vi "Init.vi"(8 "error in (no error)":errorcluster, 11 "reference in":refnum<class "Test_Base.lvclass">) -> (0 "error out":errorcluster, 3 "reference out":refnum<class "Test_Base.lvclass">)   [LabVIEW 2022 SP3, in "Test_Base.lvlib" / "Test_Base.lvclass"]
uses:
  Test_Base.lvclass
  Components/ViPER.lvlibp/ViPER.lvclass
  Components/TestView_Base.lvlibp/TestView_Base.lvclass
  Components/MES_Base.lvlibp/MES_Base.lvclass
  C:/Projects/Medulla/ViPER/Examples/Flux_Capacitor_Tester/Components/ViPER.lvlibp/ViPER.lvclass
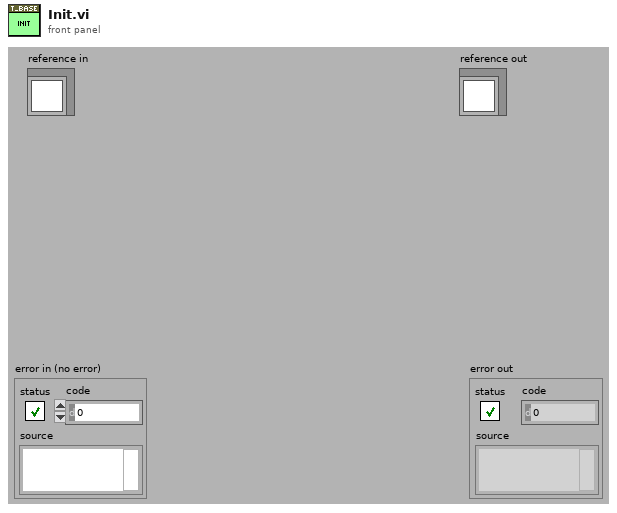
[diagram p1: front panel]
types:
  T1 = typedef "Test_Base.lvlib/Test_Base.lvclass/ObjectAttributes.ctl" = cluster{"Config":T2, "UUTIndex":i32, "Serial":string, "Batch":string, "MES":refnum<class "MES_Base.lvclass">, "TestView":refnum<class "TestView_Base.lvclass">, "LoggedIn":bool, "Abort":bool}
  T2 = typedef "Test_Base.lvlib/Test_Base.lvclass/Config.ctl" = cluster{"ContinueOnFail":bool}
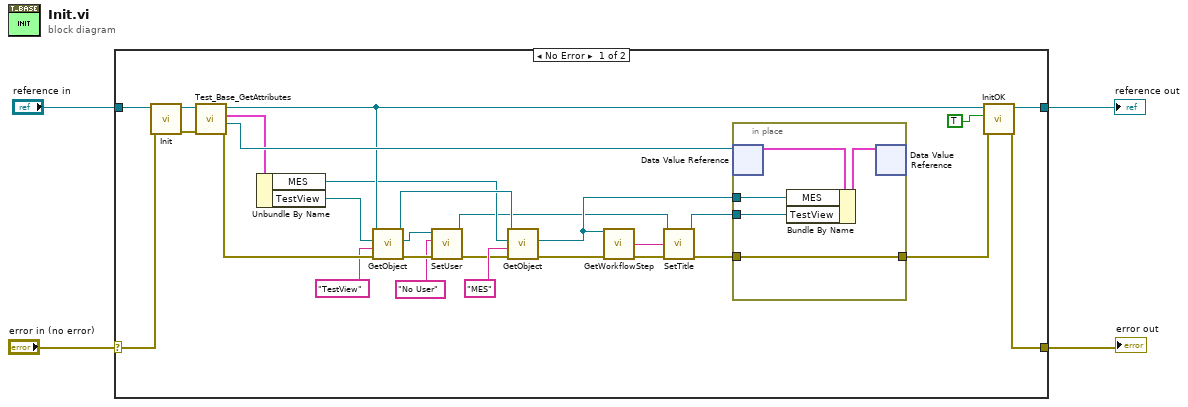
[diagram p0: block diagram]
diagram:
  n1 = case shown="No Error" "error in (no error)" {
    selector: "error in (no error)" -> [w31 w39]
    tunnel: [w24 w39] -> w3
    tunnel: [w27 w38] -> w1
    tunnel: "reference in" -> [w32 w38]
    frame No Error {
      n2 = call-parent "Init.vi"("error in (no error)"=w31, "reference in"=w32) -> ("error out"=w29:errorcluster, "reference out"=w30:refnum<class "Test_Base.lvclass">)  [unwired: 8 in]
      n3 = call "Test_Base_GetAttributes.vi"("error in (no error)"=w29, "reference in"=w30) -> ("error out"=w23:errorcluster, "DataRef"=w28:refnum<data-value>, "Data"=w22:T1, "reference out"=w21:refnum<class "Test_Base.lvclass">)  [unwired: 6 in]
      n4 = Unbundle By Name(w22) -> ("MES"=w18:refnum<class "MES_Base.lvclass">, "TestView"=w20:refnum<class "TestView_Base.lvclass">)
      n5 = call "GetObject.vi"("error in (no error)"=w23, "Object Name"="TestView", "Class type"=w20, "reference in"=w21) -> ("error out"=w13:errorcluster, "Object out"=w11:refnum<class "TestView_Base.lvclass">, "reference out"=w19:refnum<class "Test_Base.lvclass">)  [unwired: 5 in]
      n6 = call-dynamic "SetUser.vi"("error in (no error)"=w13, "User"="No User", "reference in"=w11) -> ("error out"=w12:errorcluster, "reference in"=w7:refnum<class "TestView_Base.lvclass">)  [unwired: 7 in]
      n7 = call "GetObject.vi"("error in (no error)"=w12, "Object Name"="MES", "Class type"=w18, "reference in"=w19) -> ("error out"=w15:errorcluster, "Object out"=w14:refnum<class "MES_Base.lvclass">)  [unwired: 5 in, 1 out]
      n8 = call-dynamic "GetWorkflowStep.vi"("reference in"=w14, "error in (no error)"=w15) -> ("Workflow Setp"=w5:string, "error out"=w9:errorcluster)  [unwired: 11 in, 1 out]
      n9 = call-dynamic "SetTitle.vi"("error in (no error)"=w9, "Title"=w5, "reference in"=w7) -> ("error out"=w8:errorcluster, "reference in"=w6:refnum<class "TestView_Base.lvclass">)  [unwired: 7 in]
      n10 = in-place {
        in-place-border: w8 -> [w37]
        in-place-border: [w37] -> w25
        in-place-border: w6 -> [w34]
        in-place-border: w14 -> [w33]
        n11 = in-place-dvr #1(w28) -> (w36:T1)  [unwired: 1 out]
        n12 = Bundle By Name(cluster=w36, "MES"=w33, "TestView"=w34) -> (w35:T1)
        n13 = in-place-dvr #1(w35) -> ()  [unwired: 2 out]
      }
      n14 = call "InitOK.vi"("error in (no error)"=w25, "Init OK?"=TRUE, "reference in"=w21) -> ("error out"=w24:errorcluster, "reference out"=w27:refnum<class "Test_Base.lvclass">)  [unwired: 7 in]
    }
    frame Error {
    }
  }
  "error out" <- w3
  "reference out" <- w1
